vi "type.vi"(8 "error in (no error)":errorcluster, 11 "midi-file-event in":refnum<class "midi-file-event.lvclass">) -> (0 "error out":errorcluster, 2 "type name":string, 3 "midi-file-event out":refnum<class "midi-file-event.lvclass">)   [LabVIEW 2020, in "midi-file-event.lvclass"]
uses:
  midi-file-event.lvclass
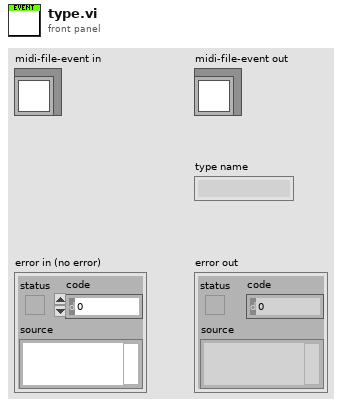
[diagram p1: front panel]
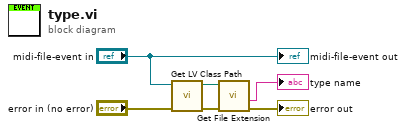
[diagram p0: block diagram]
diagram:
  n1 = call <vilib>:"Get LV Class Path.vi"("error in (no error)"="error in (no error)", "object"="midi-file-event in") -> ("error out"=w4:errorcluster, "class path"=w6:path)  [unwired: 8 in]
  n2 = call <vilib>:"Get File Extension.vi"("error in (no error)"=w4, "file"=w6) -> ("error out"=→"error out":errorcluster, "filename without extension"=→"type name":string)  [unwired: 5 in, 3 out]
  "midi-file-event out" <- "midi-file-event in"
